vi "Main.vi"() -> ()   [LabVIEW 2021]
doc: "Use this template to build a simple state machine design pattern. Each state executes code and determines which state to transition to."
uses:
  controls/State.ctl
  controls/Data.ctl
  vmmso/vmmso.lvlib
panel:
  in  "Amplitude":dbl=2000.0
  in  "Bias":dbl
  in  "Freq":dbl=1000.0
  in  "Wave Style":u16(ring) items=["Sine", "Square", "Ramp"]
  out "Is Data Ready？":bool
  out "ReadVoltageData Return":u32
  out "Voltage Wave":dbl[][](graph)
  out "Capture Return":i32
  out "Device is OK?":bool
  out "Support Samples":u32[](array[numeric])
  in  "Exit":bool
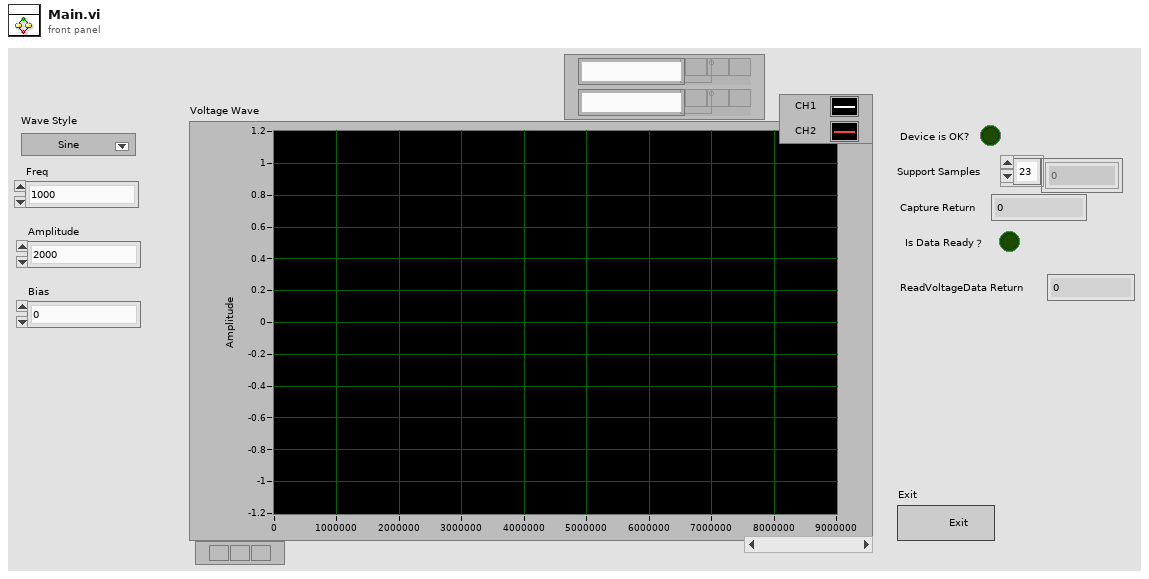
[diagram p1: front panel]
types:
  T1 = typedef "Data.ctl" = cluster{"Boolean <Replace Me>":bool, "String <Replace Me>":string, "Numeric <Replace Me>":dbl}
  T2 = typedef "State.ctl" = enum16{"Initialize", "Wait for UsbIn", "Init Osc and Dds", "Wait for Event", "Capture", "Read Voltage", "Exit"}
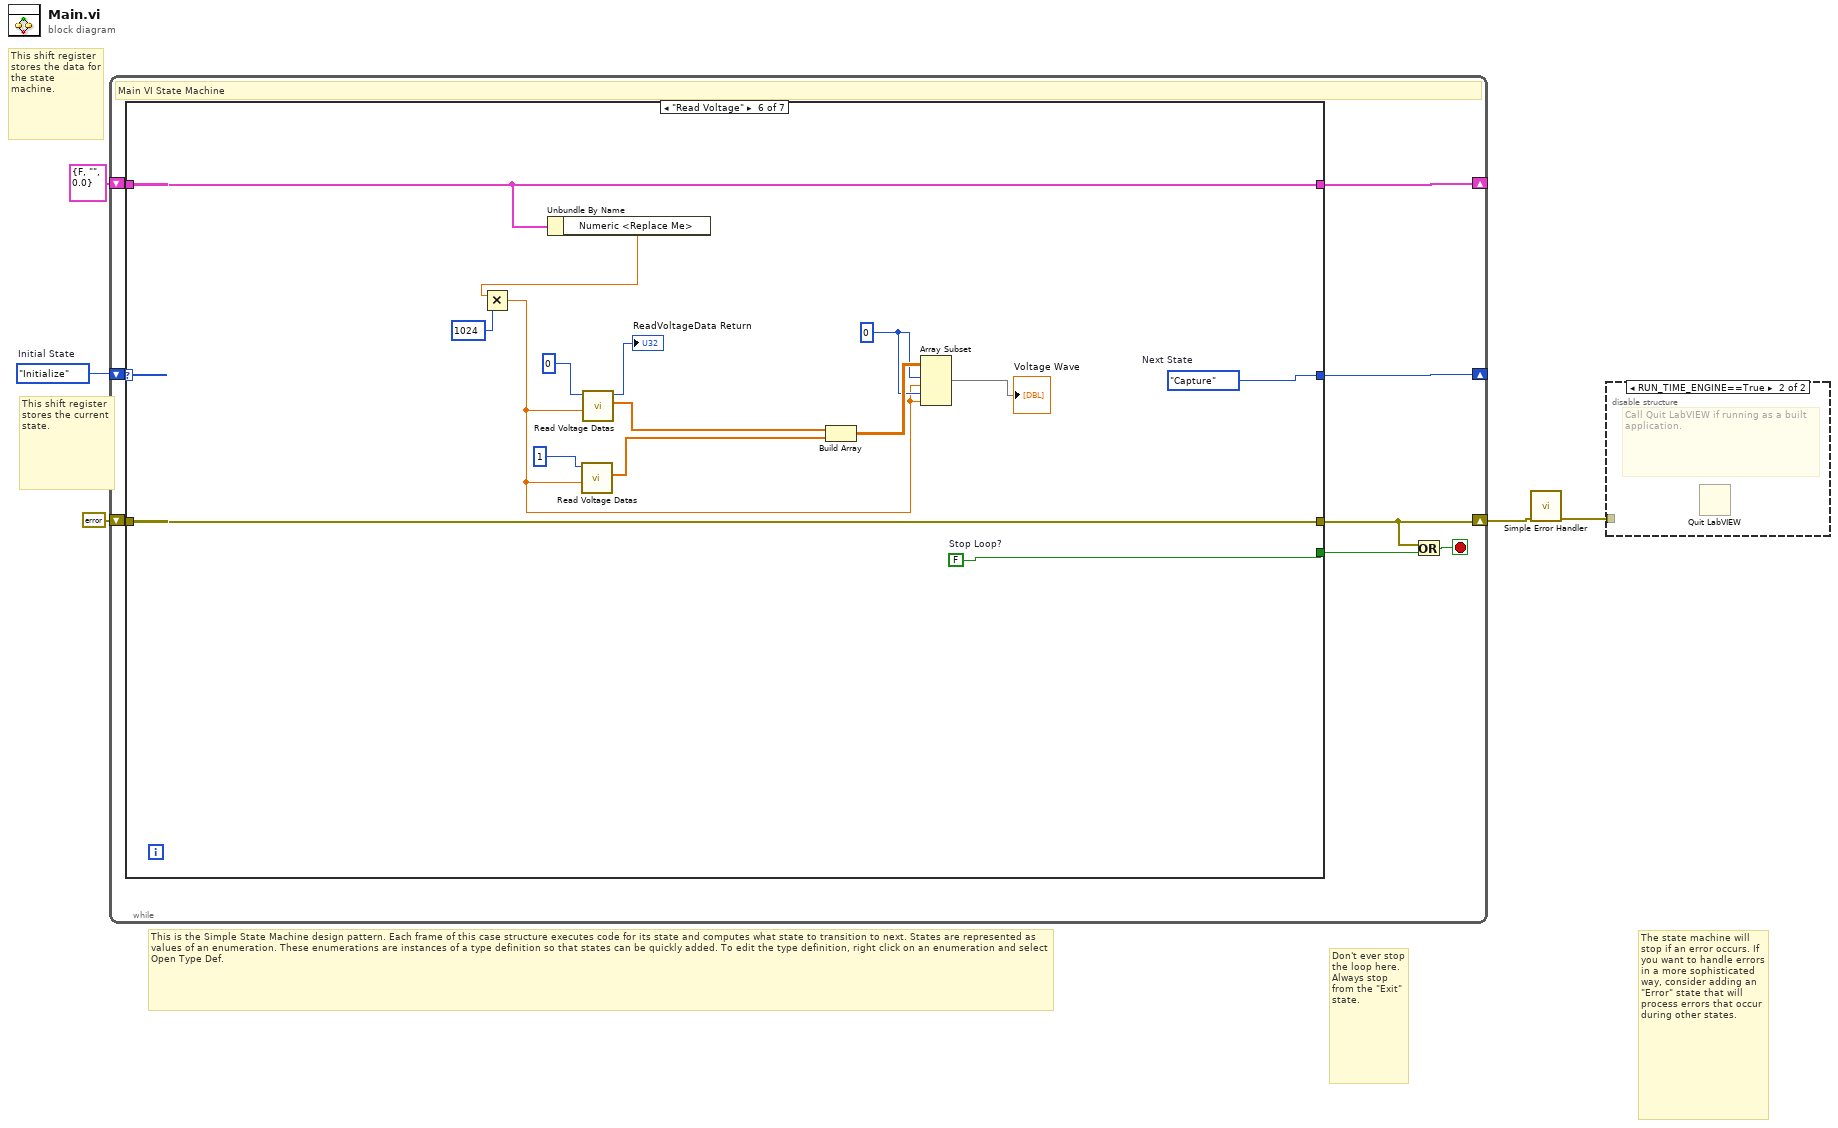
[diagram p0: block diagram]
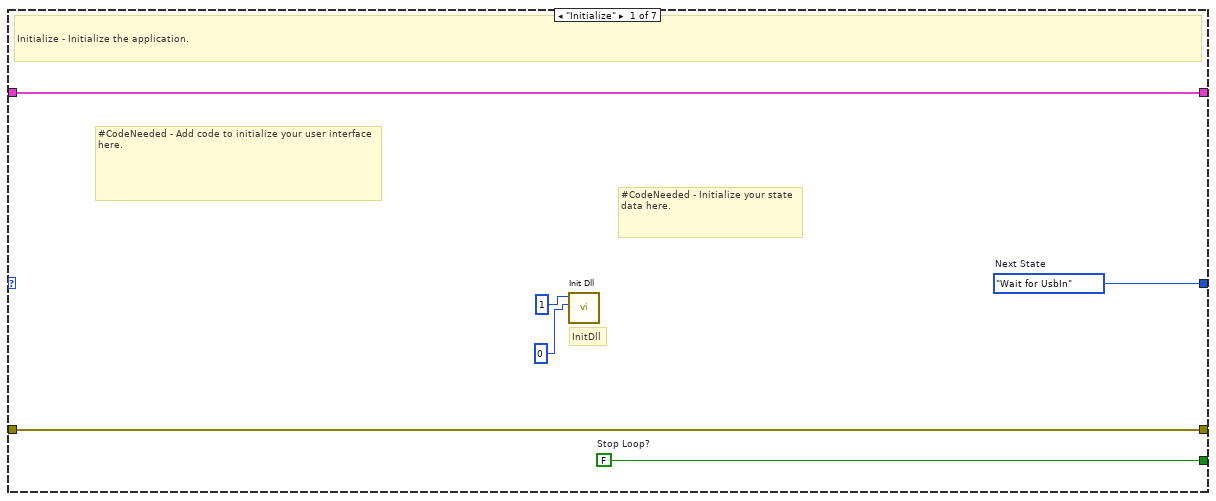
[diagram p3: hidden frame]
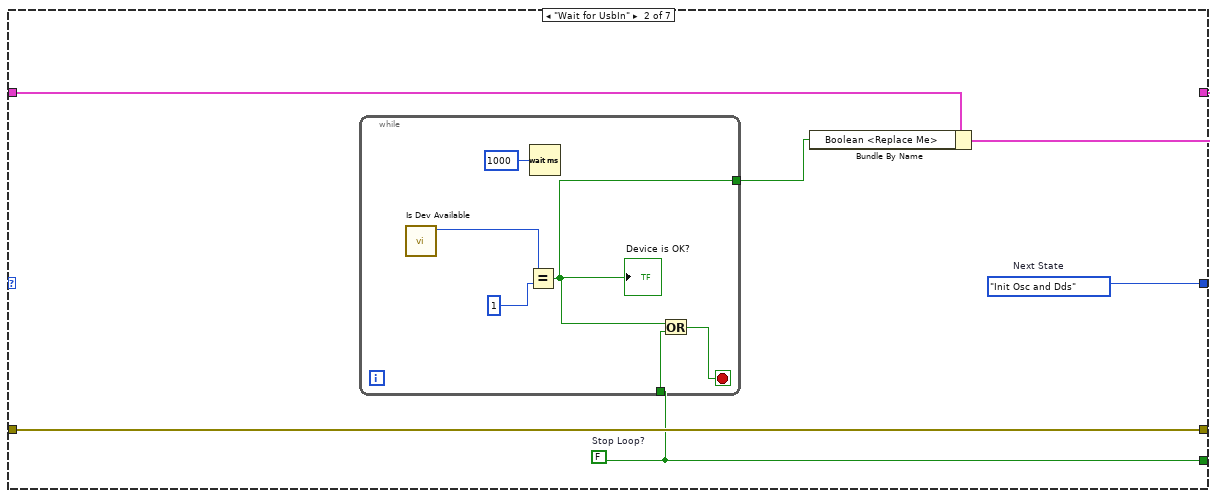
[diagram p4: hidden frame]
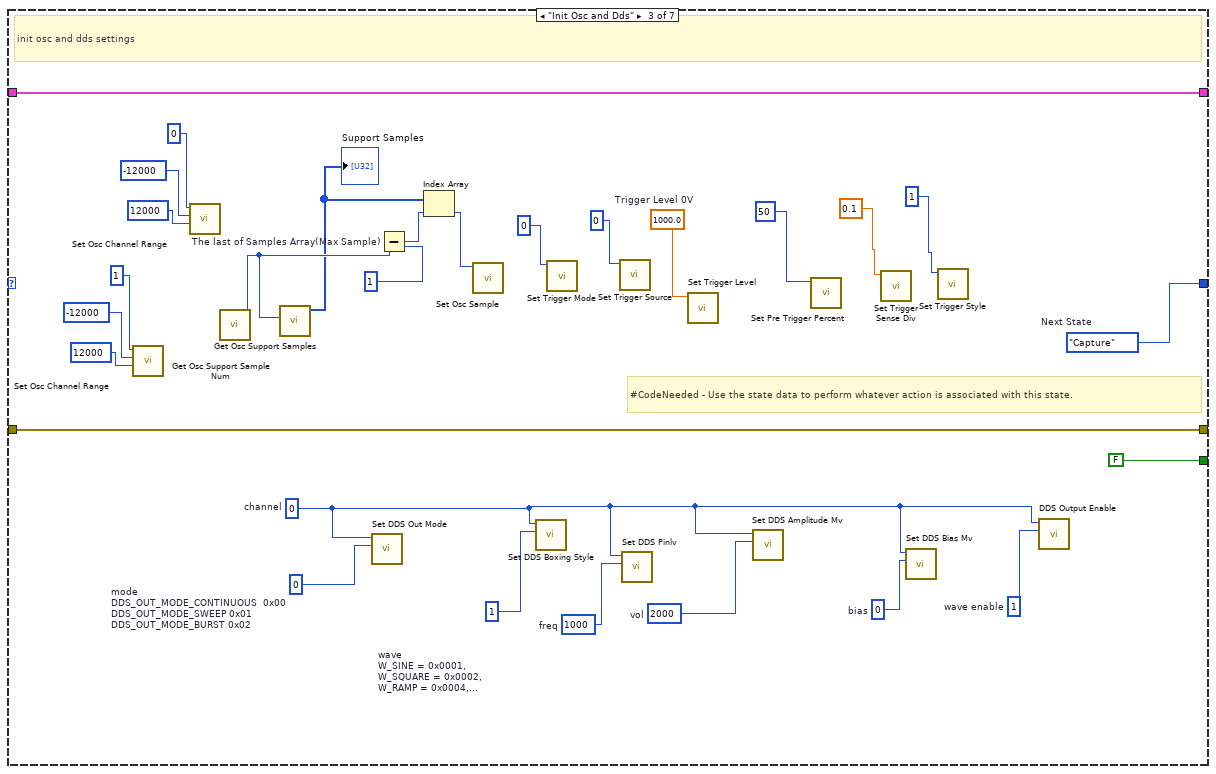
[diagram p5: hidden frame]
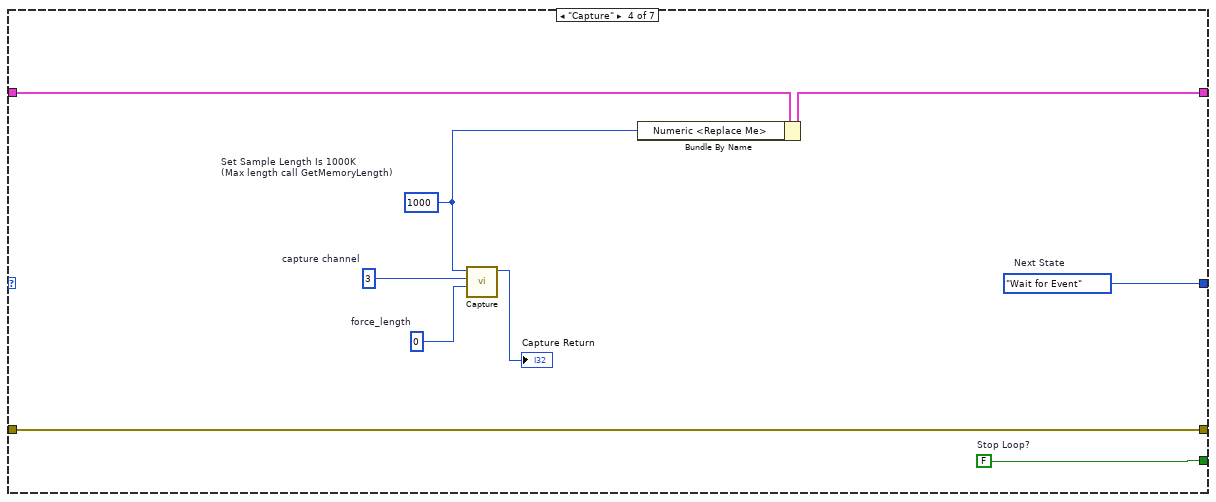
[diagram p6: hidden frame]
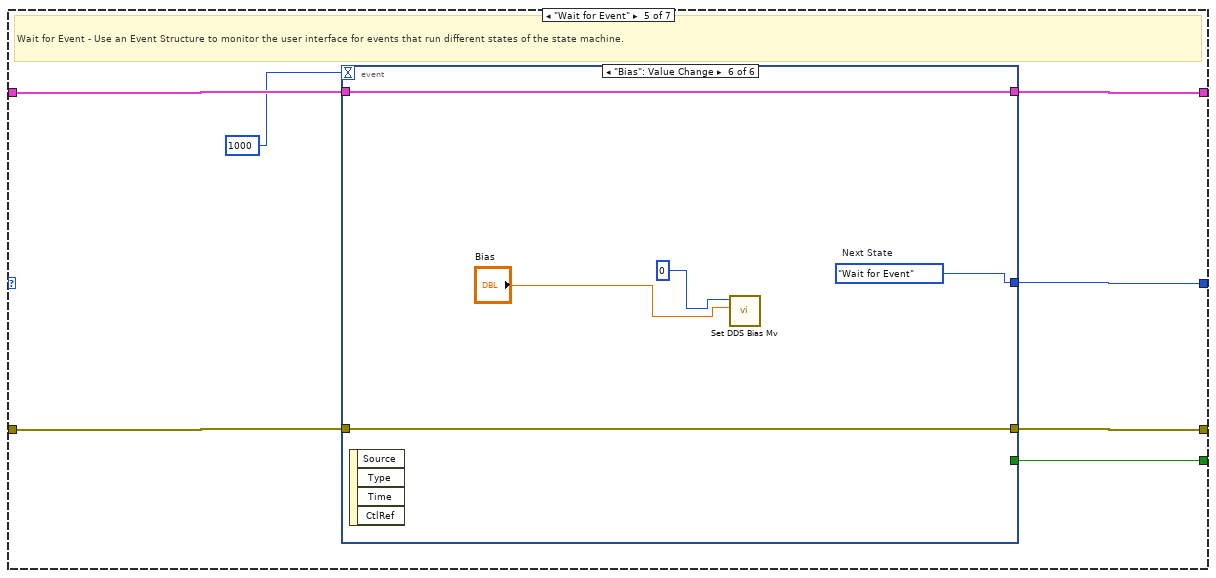
[diagram p7: hidden frame]
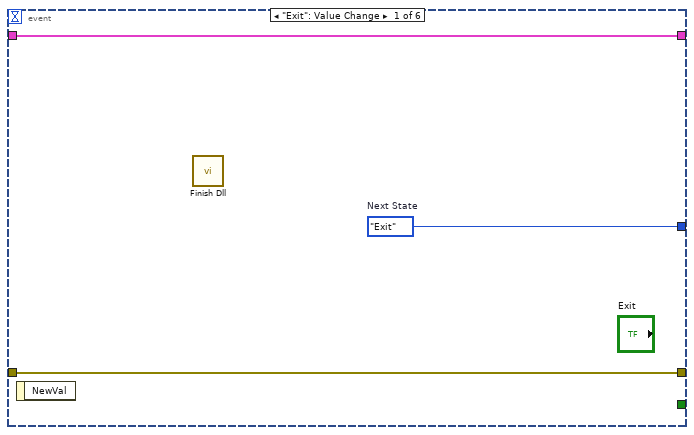
[diagram p8: hidden frame]
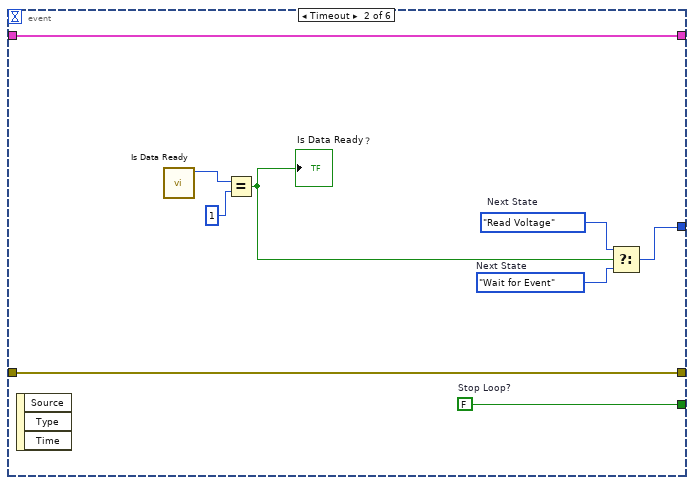
[diagram p9: hidden frame]
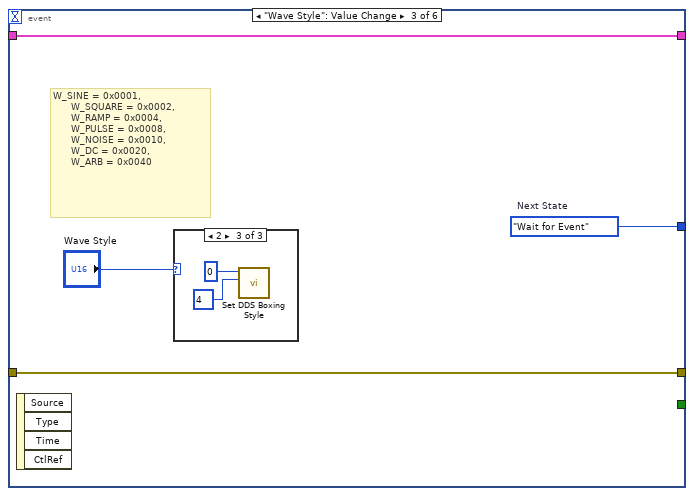
[diagram p10: hidden frame]
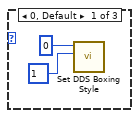
[diagram p11: hidden frame]
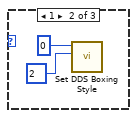
[diagram p12: hidden frame]
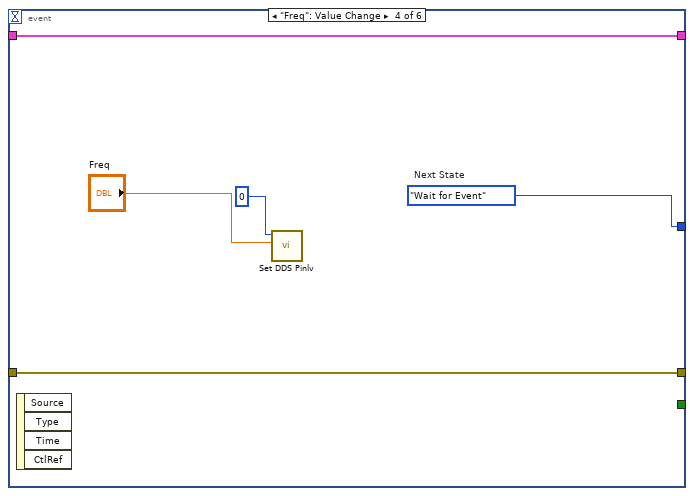
[diagram p13: hidden frame]
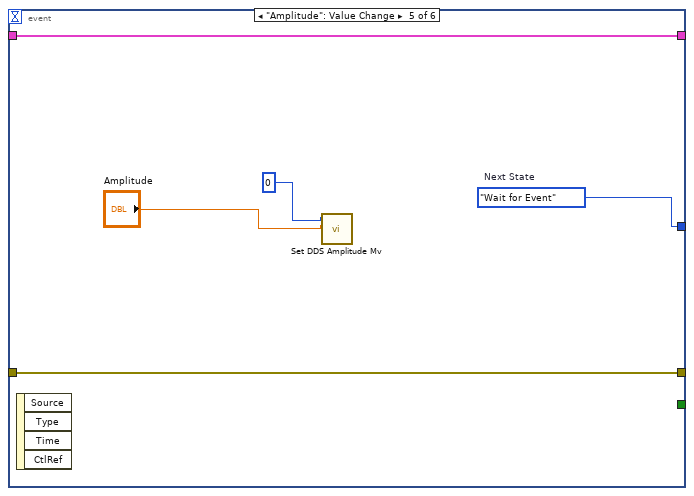
[diagram p14: hidden frame]
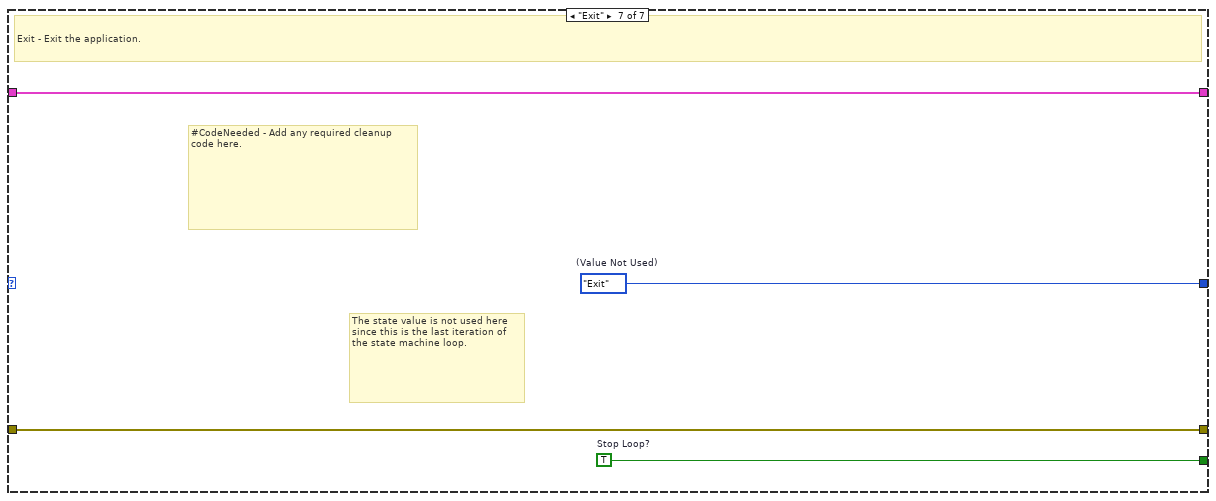
[diagram p15: hidden frame]
diagram:
  w5 = State."Initialize"  # Initial State
  # "Don't ever stop the loop here. Always stop from the \"Exit\" state."
  # "The state machine will stop if an error occurs. If you want to handle errors in a more sophisticated way, consider adding an \"Error\" state that will process errors that occur during other states."
  # "This shift register stores the data for the state machine."
  # "This is the Simple State Machine design pattern. Each frame of this case structure executes code for its state and computes what state to transition to next. States are represented as values of an enumeration. These enumerations are instances of a type definition so that states can be quickly added. To edit the type definition, right click on an enumeration and select Open Type Def."
  # "This shift register stores the current state."
  n1 = while {
    shift-right: [w12] -> _
    shift-left: w5 -> [w13]
    shift-right: [w10] -> _
    shift-left: T1 {"Boolean <Replace Me>"=FALSE, "String <Replace Me>"="", "Numeric <Replace Me>"=0.0} ("Data") -> [w11]
    shift-right: [w7] -> w2
    shift-left: errorcluster {"status"=FALSE, "code"=0, "source"=""} ("error constant") -> [w9]
    stop <- w8 stop-if-true
    # "Main VI State Machine"
    n2 = case shown="\"Read Voltage\"" w13 {
      tunnel: [w19 w24 w59 w67 w75 w125 w131] -> w12
      tunnel: w11 -> [w14 w22 w57 w62 w74 w121 w130]
      tunnel: [w14 w21 w57 w61 w73 w121 w130] -> w10
      tunnel: w9 -> [w17 w25 w56 w68 w72 w127 w128]
      tunnel: [w17 w25 w56 w68 w71 w127 w128] -> w7
      tunnel: [w18 w23 FALSE ("Stop Loop?") w66 w70 w126 w129] -> w6
      frame "Initialize" {
        w18 = FALSE  # Stop Loop?
        w19 = State."Wait for UsbIn"  # Next State
        # "InitDll"
        # "#CodeNeeded - Initialize your state data here."
        # "#CodeNeeded - Add code to initialize your user interface here."
        # "Initialize - Initialize the application."
        n3 = call "Init Dll.vi"("en_hard_watchdog"=0 ("channel"), "en_log"=1 ("channel")) -> ()  [unwired: 9 in, 1 out]
      }
      frame "Wait for UsbIn" {
        w24 = State."Init Osc and Dds"  # Next State
        w23 = FALSE  # Stop Loop?
        n4 = while {
          tunnel: w23 -> [w29]
          tunnel: [w26] -> w20
          stop <- w28 stop-if-true
          n5 = call "Is Dev Available.vi"() -> ("function return"=w27:i32)  [unwired: 11 in]
          n6 = Equal?(x=w27, y=1 ("channel")) -> (x = y?=w26:bool)
          "Device is OK?" <- w26
          n7 = Wait (ms)(milliseconds to wait=u32 1000 ("等待时间（毫秒）")) -> ()  [unwired: 1 out]
          n8 = Or(x=w26, y=w29) -> (x .or. y?=w28:bool)
        }
        n9 = Bundle By Name(cluster=w22, "Boolean <Replace Me>"=w20) -> (w21:T1)
      }
      frame "Init Osc and Dds" {
        w35 = i8 0  # mode DDS_OUT_MODE_CONTINUOUS  0x00 DDS_OUT_MODE_SWEEP 0x01 DDS_OUT_MODE_BURST 0x02
        w37 = i8 1  # wave enable
        w39 = u32 0  # bias
        w38 = u32 2000  # vol
        w40 = u32 1000  # freq
        w41 = i8 1  # wave  W_SINE = 0x0001,  W_SQUARE = 0x0002,  W_RAMP = 0x0004,  W_PULSE = 0x0008,  W_NOISE = 0x0010,  W_DC = 0x0020,  W_ARB = 0x0040
        w36 = i8 0  # channel
        w51 = sgl 1000.0  # Trigger Level 0V
        w59 = State."Capture"  # Next State
        # "#CodeNeeded - Use the state data to perform whatever action is associated with this state."
        # "init osc and dds settings"
        n10 = call "Set Osc Channel Range.vi"("maxmv"=12000 ("minmv"), "minmv"=-12000, "channel"=1) -> ()  [unwired: 8 in, 1 out]
        n11 = call "Set Osc Channel Range.vi"("maxmv"=12000 ("minmv"), "minmv"=-12000, "channel"=0) -> ()  [unwired: 8 in, 1 out]
        n12 = call "Get Osc Support Sample Num.vi"() -> ("function return"=w47:i32)  [unwired: 11 in]
        n13 = call "Get Osc Support Samples.vi"("maxnum"=w47) -> ("sample out"=w44:u32[])  [unwired: 9 in, 1 out]
        "Support Samples" <- w44
        n14 = call "Set DDS Out Mode.vi"("out_mode"=w35, "channel_index"=w36) -> ()  [unwired: 10 in]
        n15 = Subtract "The last of Samples Array(Max Sample)"(x=w47, y=1 ("front")) -> (x-y=w49:i32)
        n16 = Index Array(array=w44, index=w49) -> (element=w50:u32)
        n17 = call "Set Osc Sample.vi"("sample"=w50) -> ()  [unwired: 10 in, 1 out]
        n18 = call "Set DDS Boxing Style.vi"("boxing"=w41, "channel_index"=w36) -> ()  [unwired: 10 in]
        n19 = call "Set Trigger Mode.vi"("mode"=0 ("front")) -> ()  [unwired: 11 in]
        n20 = call "Set Trigger Source.vi"("source"=0 ("front")) -> ()  [unwired: 11 in]
        n21 = call "Set DDS Pinlv.vi"("pinlv"=w40, "channel_index"=w36) -> ()  [unwired: 10 in]
        n22 = call "Set Trigger Level.vi"("level"=w51) -> ()  [unwired: 11 in]
        n23 = call "Set DDS Amplitude Mv.vi"("amplitdude"=w38, "channel_index"=w36) -> ()  [unwired: 10 in]
        n24 = call "Set Pre Trigger Percent.vi"("front"=50) -> ()  [unwired: 11 in]
        n25 = call "Set Trigger Sense Div.vi"("sense"=0.1) -> ()  [unwired: 11 in]
        n26 = call "Set DDS Bias Mv.vi"("bias"=w39, "channel_index"=w36) -> ()  [unwired: 10 in]
        n27 = call "Set Trigger Style.vi"("style"=u32 1) -> ()  [unwired: 11 in]
        n28 = call "DDS Output Enable.vi"("enable"=w37, "channel_index"=w36) -> ()  [unwired: 10 in]
      }
      frame "Capture" {
        w63 = i8 0  # force_length
        w60 = u32 1000  # Set Sample Length Is 1000K (Max length call GetMemoryLength)
        w64 = i8 3  # capture channel
        w66 = FALSE  # Stop Loop?
        w67 = State."Wait for Event"  # Next State
        n29 = call "Capture.vi"("force_length"=w63, "capture_channel"=w64, "length"=w60) -> ("function return"=→"Capture Return":i32)  [unwired: 8 in]
        n30 = Bundle By Name(cluster=w62, "Numeric <Replace Me>"=w60) -> (w61:T1)
      }
      frame "Wait for Event" {
        # "Wait for Event - Use an Event Structure to monitor the user interface for events that run different states of the state machine."
        n31 = event shown="[5] \"Bias\": Value Change" {
          selector: _ -> [_ _ _ _ _ _]
          dyn-events: _ -> [_ _ _ _ _ _]
          timeout: 1000 ("y") -> [_ _ _ _ _ _]
          tunnel: [w78 w82 w88 w100 w105 w110] -> w75
          tunnel: w74 -> [w77 w87 w91 w102 w107 w112]
          tunnel: [w77 w87 w91 w102 w107 w112] -> w73
          tunnel: w72 -> [w76 w86 w90 w101 w106 w111]
          tunnel: [w76 w86 w90 w101 w106 w111] -> w71
          tunnel: [_ w83 _ _ _ _] -> w70
          event "Exit": Value Change {
            w78 = State."Exit"  # Next State
            n32 = event-data() -> ()  [unwired: 1 in, 1 out]
            n33 = call "Finish Dll.vi"() -> ()  [unwired: 11 in, 1 out]
          }
          event Timeout {
            w79 = State."Wait for Event"  # Next State
            w83 = FALSE  # Stop Loop?
            w80 = State."Read Voltage"  # Next State
            n34 = event-data() -> ()  [unwired: 1 in, 3 out]
            n35 = call "Is Data Ready.vi"() -> ("function return"=w85:i32)  [unwired: 11 in]
            n36 = Equal?(x=w85, y=1) -> (x = y?=w81:bool)
            "Is Data Ready？" <- w81
            n37 = Select(t=w80, s=w81, f=w79) -> (s? t:f=w82:T2)
          }
          event "Wave Style": Value Change {
            w88 = State."Wait for Event"  # Next State
            # "W_SINE = 0x0001, \n\t\t\t\t\t\tW_SQUARE = 0x0002, \n\t\t\t\t\t\tW_RAMP = 0x0004, \n\t\t\t\t\t\tW_PULSE = 0x0008, \n\t\t\t\t\t\tW_NOISE = 0x0010, \n\t\t\t\t\t\tW_DC = 0x0020, \n\t\t\t\t\t\tW_ARB = 0x0040"
            n38 = event-data() -> ()  [unwired: 1 in, 4 out]
            n39 = case shown="2" "Wave Style" {
              frame 0, Default {
                n40 = call "Set DDS Boxing Style.vi"("boxing"=1 ("y"), "channel_index"=0 ("y")) -> ()  [unwired: 10 in]
              }
              frame 1 {
                n41 = call "Set DDS Boxing Style.vi"("boxing"=2 ("y"), "channel_index"=0 ("y")) -> ()  [unwired: 10 in]
              }
              frame 2 {
                n42 = call "Set DDS Boxing Style.vi"("boxing"=4 ("y"), "channel_index"=0 ("y")) -> ()  [unwired: 10 in]
              }
            }
          }
          event "Freq": Value Change {
            w100 = State."Wait for Event"  # Next State
            n43 = event-data() -> ()  [unwired: 1 in, 4 out]
            n44 = call "Set DDS Pinlv.vi"("pinlv"="Freq", "channel_index"=0 ("y")) -> ()  [unwired: 10 in]
          }
          event "Amplitude": Value Change {
            w105 = State."Wait for Event"  # Next State
            n45 = event-data() -> ()  [unwired: 1 in, 4 out]
            n46 = call "Set DDS Amplitude Mv.vi"("amplitdude"="Amplitude", "channel_index"=0 ("y")) -> ()  [unwired: 10 in]
          }
          event "Bias": Value Change {
            w110 = State."Wait for Event"  # Next State
            n47 = event-data() -> ()  [unwired: 1 in, 4 out]
            n48 = call "Set DDS Bias Mv.vi"("bias"="Bias", "channel_index"=0 ("y")) -> ()  [unwired: 10 in]
          }
        }
      }
      frame "Read Voltage" {
        w114 = i8 0 ("channel")
        w125 = State."Capture"  # Next State
        w126 = FALSE  # Stop Loop?
        n49 = Unbundle By Name(w121) -> ("Numeric <Replace Me>"=w120:dbl)
        n50 = Multiply(x=w120, y=1024) -> (x*y=w113:dbl)
        n51 = call "Read Voltage Datas.vi"("length"=w113, "channel"=i8 1) -> ("buffer out"=w117:dbl[])  [unwired: 8 in, 1 out]
        n52 = call "Read Voltage Datas.vi"("length"=w113, "channel"=i8 0) -> ("buffer out"=w118:dbl[], "function return"=→"ReadVoltageData Return":u32)  [unwired: 8 in]
        n53 = Build Array(w118, w117) -> (w116:dbl[][])
        n54 = Array Subset(array=w116, index (row)=w114, length (row)=w113, index (col)=w114, length (col)=w113) -> (→"Voltage Wave":dbl[][])
      }
      frame "Exit" {
        w129 = TRUE  # Stop Loop?
        w131 = State."Exit"  # (Value Not Used)
        # "#CodeNeeded - Add any required cleanup code here."
        # "The state value is not used here since this is the last iteration of the state machine loop."
        # "Exit - Exit the application."
      }
    }
    n55 = Or(x=w7, y=w6) -> (x .or. y?=w8:bool)
  }
  n56 = call <vilib>:"Simple Error Handler.vi"("error in (no error)"=w2) -> ("error out"=w1:errorcluster)  [unwired: 4 in, 4 out]
  n57 = disable-structure shown="RUN_TIME_ENGINE==True" {
    disable-tunnel: w1 -> [_ _]
    frame condition #0 (active) {
    }
    frame condition #1 {
      # "Call Quit LabVIEW if running as a built application."
      n58 = Quit LabVIEW() -> ()  [unwired: 1 in]
    }
  }
